vi "Main.vi"() -> ()   [LabVIEW 2018]
panel:
  out "Waiting Lights":T1
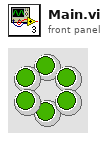
[diagram p1: front panel]
types:
  T1 = cluster{"wait 1":bool, "wait 2":bool, "wait 3":bool, "wait 4":bool, "wait 5":bool, "wait 6":bool}
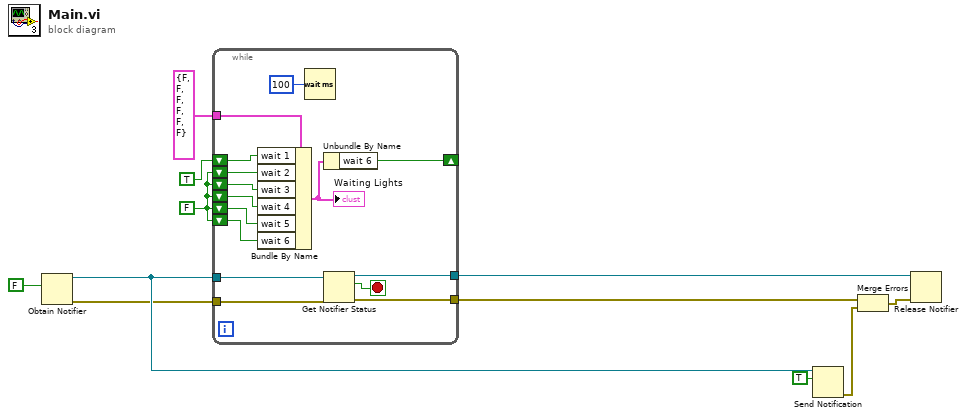
[diagram p0: block diagram]
diagram:
  w10 = FALSE ("wait 1")
  n1 = Obtain Notifier(notification data type=FALSE ("wait 1")) -> (notifier out=w6:refnum<notifier>, error out=w5:errorcluster)  [unwired: 3 in, 1 out]
  n2 = while {
    tunnel: T1 {"wait 1"=FALSE, "wait 2"=FALSE, "wait 3"=FALSE, "wait 4"=FALSE, "wait 5"=FALSE, "wait 6"=FALSE} ("Waiting Lights") -> [w26]
    shift-right: [w18] -> _
    shift-left: TRUE ("wait 1") -> [w25]
    shift-left: w10 -> [w24]
    shift-left: w10 -> [w23]
    shift-left: w10 -> [w22]
    shift-left: w10 -> [w21]
    shift-left: w10 -> [w20]
    tunnel: w6 -> [w16]
    tunnel: [w15] -> w7
    tunnel: w5 -> [w13]
    tunnel: [w12] -> w3
    stop <- w14 stop-if-true
    n3 = Bundle By Name(cluster=w26, "wait 1"=w25, "wait 2"=w24, "wait 3"=w23, "wait 4"=w22, "wait 5"=w21, "wait 6"=w20) -> (w19:T1)
    "Waiting Lights" <- w19
    n4 = Wait (ms)(milliseconds to wait=u32 100) -> ()  [unwired: 1 out]
    n5 = Unbundle By Name(w19) -> ("wait 6"=w18:bool)
    n6 = Get Notifier Status(notifier=w16, error in (no error)=w13) -> (notifier out=w15:refnum<notifier>, current notification=w14:bool, error out=w12:errorcluster)  [unwired: 2 out]
  }
  n7 = Send Notification(notification=TRUE, notifier=w6) -> (error out=w2:errorcluster)  [unwired: 1 in, 1 out]
  n8 = Merge Errors(w3, w2) -> (w4:errorcluster)
  n9 = Release Notifier(notifier=w7, error in (no error)=w4) -> ()  [unwired: 1 in, 3 out]
